vi "Test LogRecord Init.vi"(8 "error in":errorcluster) -> (0 "error out":errorcluster)   [LabVIEW 2016, in "UT_LogRecord.lvlib"]
doc: "Test the initialization and Getter-methods."
uses:
  UT_LogRecord.lvlib
  Source/HSE-Logger/LogLevel.ctl
  Source/HSE-Logger/LogRecord/LogRecord.lvclass/LogRecord.ctl
  <vilib>/addons/_JKI Toolkits/Caraya/classes/Test/Test.lvclass
  Source/HSE-Logger/hse-logger.lvlib
  Source/HSE-Logger/LogRecord/LogRecord.lvclass
  <vilib>/addons/_JKI Toolkits/Caraya/classes/Assert/Assert.lvclass
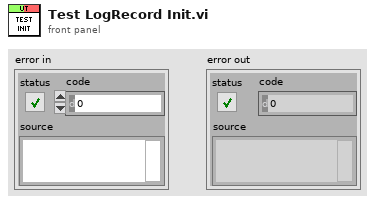
[diagram p1: front panel]
types:
  T1 = typedef "hse-logger.lvlib/LogLevel.ctl" = enum16{"DEBUG", "INFO", "WARNING", "ERROR", "CRITICAL"}
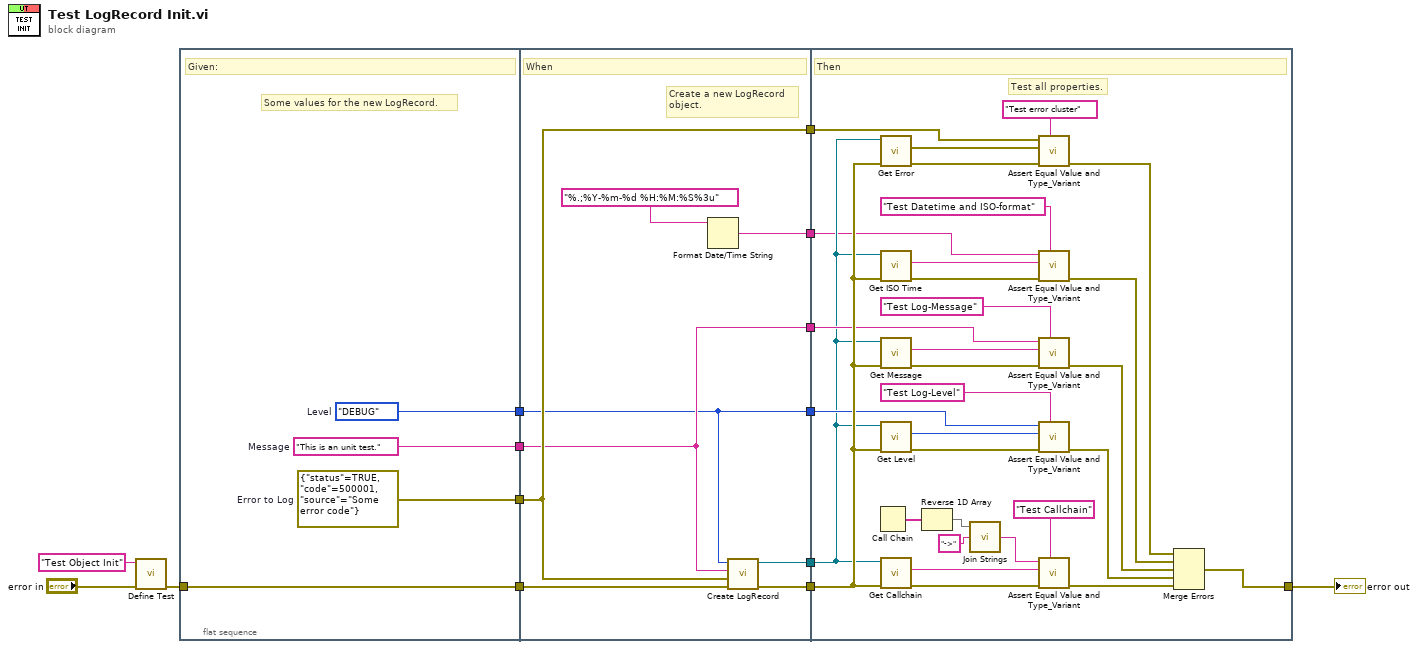
[diagram p0: block diagram]
diagram:
  n1 = call <vilib>:"Define Test.vi"("error in (no error)"="error in", "Label (VI Title)"="Test Object Init") -> ("error out"=w10:errorcluster)  [unwired: 8 in, 1 out]
  n2 = flat-sequence {
    tunnel: w10 -> [w17]
    tunnel: [w17] -> w14
    tunnel: [w16] -> w6
    tunnel: [w15] -> w5
    tunnel: [w18] -> w9
    tunnel: w14 -> [w25]
    tunnel: [w24] -> w13
    tunnel: w6 -> [w21]
    tunnel: w5 -> [w22]
    tunnel: w9 -> [w26]
    tunnel: [w23] -> w4
    tunnel: [w26] -> w8
    tunnel: [w22] -> w3
    tunnel: [w21] -> w2
    tunnel: [w19] -> w1
    tunnel: [w48] -> w12
    tunnel: w2 -> [w36]
    tunnel: w3 -> [w39]
    tunnel: w8 -> [w56]
    tunnel: w4 -> [w34]
    tunnel: w13 -> [w51]
    tunnel: w1 -> [w29]
    frame #0 {
      w18 = errorcluster {"status"=TRUE, "code"=500001, "source"="Some error code"}  # Error to Log
      w15 = "This is an unit test."  # Message
      w16 = LogLevel."DEBUG"  # Level
      # "Some values for the new LogRecord."
      # "Given:"
    }
    frame #1 {
      # "Create a new LogRecord\nobject."
      # "When"
      n3 = Format Date/Time String(time format string (%c)="%.;%Y-%m-%d %H:%M:%S%3u") -> (date/time string=w19:string)  [unwired: 2 in]
      n4 = call "Create LogRecord.vi"("error in"=w25, "Error to Log"=w26, "Message"=w22, "Level"=w21) -> ("error out"=w24:errorcluster, "LogRecord out"=w23:refnum<class "LogRecord.lvclass">)  [unwired: 6 in]
    }
    frame #2 {
      # "Test all properties."
      # "Then"
      n5 = Call Chain() -> (call chain=w28:string[])
      n6 = call "Get Error.vi"("error in"=w51, "LogRecord in"=w34) -> ("error out"=w54:errorcluster, "Error"=w57:errorcluster)  [unwired: 7 in, 1 out]
      n7 = call "Get ISO Time.vi"("error in"=w51, "LogRecord in"=w34) -> ("error out"=w55:errorcluster, "ISO Time"=w41:string)  [unwired: 7 in, 1 out]
      n8 = call "Get Message.vi"("error in"=w51, "LogRecord in"=w34) -> ("error out"=w53:errorcluster, "Message"=w40:string)  [unwired: 7 in, 1 out]
      n9 = call "Get Level.vi"("error in"=w51, "LogRecord in"=w34) -> ("error out"=w52:errorcluster, "Level"=w35:T1)  [unwired: 7 in, 1 out]
      n10 = call "Get Callchain.vi"("error in"=w51, "LogRecord in"=w34) -> ("error out"=w50:errorcluster, "Callchain"=w32:string)  [unwired: 7 in, 1 out]
      n11 = Reverse 1D Array(array=w28) -> (reversed array=w27:string[])
      n12 = call <vilib>:"Join Strings.vi"("Separator (,)"="->", "Strings In"=w27) -> ("String"=w31:string)  [unwired: 1 in]
      n13 = call <vilib>:"Assert Equal Value and Type_Variant.vi"("Label"="Test error cluster", "error in (no error)"=w54, "Y"=w57, "X"=w56) -> ("error out"=w44:errorcluster)  [unwired: 6 in, 1 out]
      n14 = call <vilib>:"Assert Equal Value and Type_Variant.vi"("Label"="Test Datetime and ISO-format", "error in (no error)"=w55, "Y"=w41, "X"=w29) -> ("error out"=w45:errorcluster)  [unwired: 6 in, 1 out]
      n15 = call <vilib>:"Assert Equal Value and Type_Variant.vi"("Label"="Test Log-Message", "error in (no error)"=w53, "Y"=w40, "X"=w39) -> ("error out"=w46:errorcluster)  [unwired: 6 in, 1 out]
      n16 = call <vilib>:"Assert Equal Value and Type_Variant.vi"("Label"="Test Log-Level", "error in (no error)"=w52, "Y"=w35, "X"=w36) -> ("error out"=w47:errorcluster)  [unwired: 6 in, 1 out]
      n17 = call <vilib>:"Assert Equal Value and Type_Variant.vi"("Label"="Test Callchain", "error in (no error)"=w50, "Y"=w32, "X"=w31) -> ("error out"=w49:errorcluster)  [unwired: 6 in, 1 out]
      n18 = Merge Errors(w44, w45, w46, w47, w49) -> (w48:errorcluster)
    }
  }
  "error out" <- w12
